vi "Clear Console.vi"(8 "error in (no error)":errorcluster, 11 "Console Log in":refnum<class "Console Log.lvclass">) -> (0 "error out":errorcluster, 3 "Console Log out":refnum<class "Console Log.lvclass">)   [LabVIEW 2011, in "Console Log.lvclass"]
uses:
  Console Log.lvclass
  Console Log.lvclass/Console Log.ctl
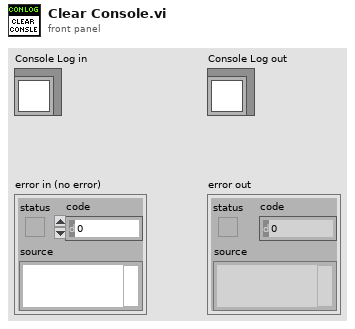
[diagram p1: front panel]
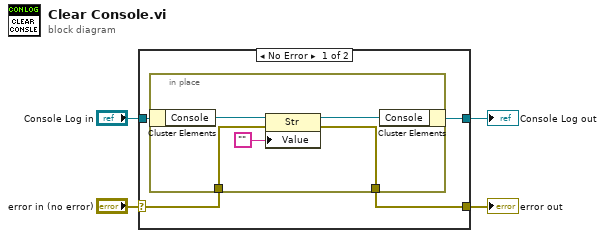
[diagram p0: block diagram]
diagram:
  n1 = case shown="No Error" "error in (no error)" {
    selector: "error in (no error)" -> [w8 w15]
    tunnel: [w7 w15] -> w3
    tunnel: [w5 w14] -> w1
    tunnel: "Console Log in" -> [w6 w14]
    frame No Error {
      n2 = in-place {
        in-place-border: w8 -> [w10]
        in-place-border: [w9] -> w7
        n3 = in-place-cluster #1(w6) -> ("Console"=w13:refnum<vi>)
        n4 = property class="Str"(reference=w13, error in=w10, "Value"="") -> (reference out=w12:refnum<vi>, error out=w9:errorcluster)
        n5 = in-place-cluster #1("Console"=w12) -> (w5:refnum<class "Console Log.lvclass">)
      }
    }
    frame Error {
    }
  }
  "error out" <- w3
  "Console Log out" <- w1
